vi "test Compare Ports Between Import and Sysdef.vi"(8 "error in":errorcluster, 11 "TestCase in":refnum<class "Refresh.lvclass">) -> (0 "error out":errorcluster, 3 "TestCase out":refnum<class "Refresh.lvclass">)   [LabVIEW 2020, in "Refresh.lvclass"]
uses:
  Refresh.lvclass
  <vilib>/addons/_JKI Toolkits/VI Tester/TestCase.llb/TestCase.lvclass
  niveristand-custom-device-testing-tools/VeriStandTestUtilities/VeriStandTestUtilities.lvlib
  Scripting/AIM/AIM ARINC 429 Scripting.lvlib
  Import/ARINC 429 Import.lvlib
  System Explorer/Implementation/Implementation.lvlib
  C:/Program Files (x86)/National Instruments/LabVIEW 2020/vi.lib/addons/_JKI Toolkits/VI Tester/TestCase.llb/TestCase.lvclass
  C:/git/ni/niveristand-aim-arinc429-custom-device/Source/Custom Device Support/Tests/Unit/Refresh/Refresh.lvclass
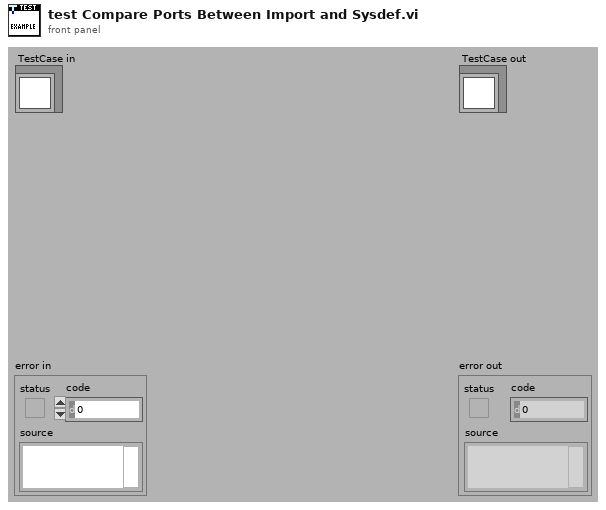
[diagram p1: front panel]
types:
  T1 = typedef "Custom Device API.lvlib/Custom Device Item Ref.ctl" = u64
  T2 = typedef "VS Channels Definition for All Labels on Hardware Channel.ctl" = cluster{"hardware channel":i32, "direction":T3, "labels":T4[], "speed":T9}
  T3 = typedef "Direction.ctl" = enum16{"Rx", "Tx"}
  T4 = typedef "VS Channels Definition for Label.ctl" = cluster{"label (Dec)":u32, "parameters":T5[], "SDI value":u8, "SDI enabled":bool, "transfer type":T8, "create timestamp":bool, "transmit period":u32}
  T5 = typedef "VS Channel Definition for Parameter.ctl" = cluster{"name":string, "unit":string, "Parameter":T6}
  T6 = typedef "Parameter Definition.ctl" = cluster{"start index":i32, "size":i32, "encoding":T7, "signed":bool, "scale multiplier":dbl, "scale offset":dbl, "default value":dbl}
  T7 = typedef "Encoding and Decoding.lvlib/Encoding.ctl" = enum16{"BNR", "BCD", "Discrete"}
  T8 = typedef "Transfer Type.ctl" = enum16{"Scheduled", "Acyclic", "Block", "Strobe"}
  T9 = typedef "Transfer Speed.ctl" = enum16{"LO (12.5 kb/s)", "HI (100 kb/s)"}
  T10 = typedef "AIM ARINC 429 System Explorer.lvlib/Implementation.lvlib/Refresh Listbox.ctl" = cluster{"Item Names":string[], "Item Symbol":T11, "Change Flag":bool}
  T11 = typedef "AIM ARINC 429 System Explorer.lvlib/Implementation.lvlib/Refresh Symbols.ctl" = enum16{"Blank", "Port", "Incoming", "Outgoing", "Label", "Word", "Parameter", "ARINC-429", "Config Files", "Channel Spec", "Item"}
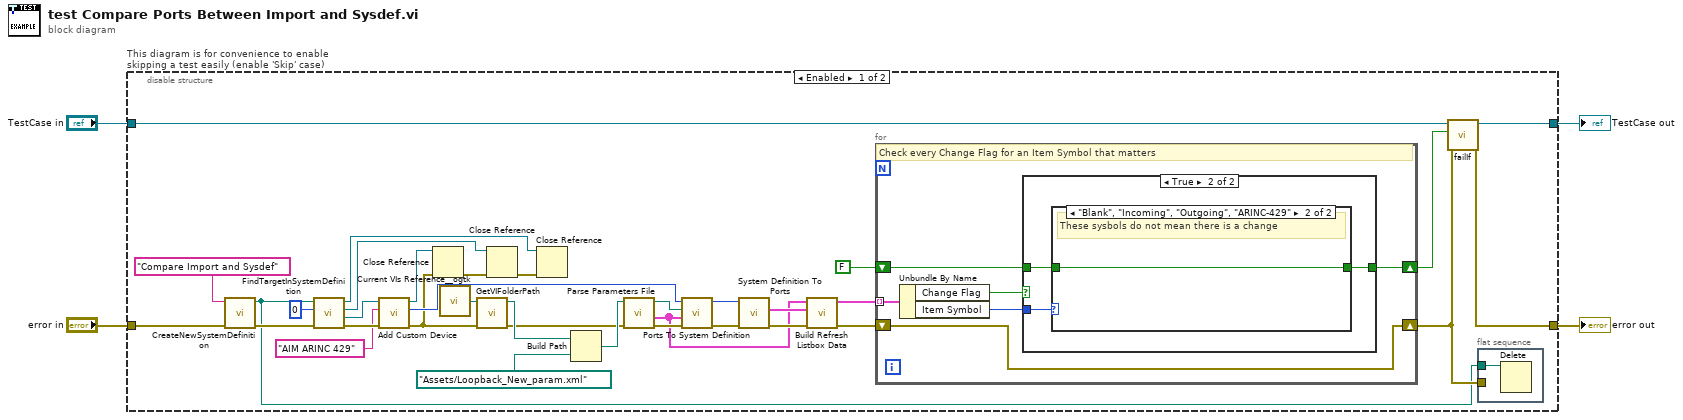
[diagram p0: block diagram]
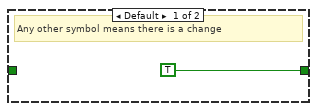
[diagram p3: hidden frame]
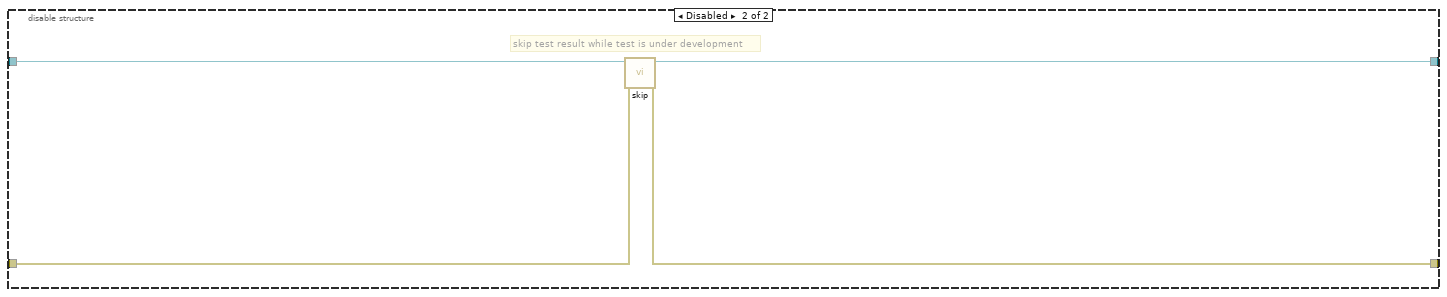
[diagram p4: hidden frame]
diagram:
  n1 = disable-structure "This diagram is for convenience to enable skipping a test easily (enable 'Skip' case)" shown="Enabled" {
    disable-tunnel: "TestCase in" -> [w25 w55]
    disable-tunnel: [w29 w56] -> w1
    disable-tunnel: [w26 w53] -> w3
    disable-tunnel: "error in" -> [w9 w54]
    frame Enabled {
      n2 = call "CreateNewSystemDefinition.vi"("error in"=w9, "System Definition Name"="Compare Import and Sysdef") -> ("error out"=w17:errorcluster, "System Definition Path"=w5:path)  [unwired: 8 in]
      n3 = call "FindTargetInSystemDefinition.vi"("error in"=w17, "target index"=0 ("index"), "system definition path"=w5) -> ("error out"=w20:errorcluster, "Target"=w19:refnum<k24>, "Root"=w13:refnum<k24>, "System Definition"=w12:refnum<k24>)  [unwired: 5 in]
      n4 = call "Add Custom Device.vi"("error in"=w20, "name"="AIM ARINC 429", "target"=w19) -> ("error out"=w8:errorcluster, "AIM ARINC 429 custom device"=w10:T1, "target out"=w16:refnum<k24>)  [unwired: 6 in]
      n5 = Close Reference(reference=w16, error in (no error)=w8) -> (error out=w14:errorcluster)
      n6 = call <userlib>:"Current VIs Reference__ogtk.vi"() -> ("Current VI's reference"=w39:refnum<vi>)  [unwired: 5 in]
      n7 = call "GetVIFolderPath.vi"("error in (no error)"=w8, "VI Reference in"=w39) -> ("error out"=w7:errorcluster, "VI Folder Path out"=w22:path)  [unwired: 8 in]
      n8 = Close Reference(reference=w13, error in (no error)=w14) -> (error out=w15:errorcluster)
      n9 = Close Reference(reference=w12, error in (no error)=w15) -> ()  [unwired: 1 out]
      n10 = Build Path(base path=w22, name or relative path=path "Assets/Loopback_New_param.xml" ("Absolute or Relative Path")) -> (appended path=w11:path)
      n11 = call "Parse Parameters File.vi"("error in"=w7, "path to XML document"=w11) -> ("error out"=w37:errorcluster, "ports"=w32:T2[], "path to XML document out"=w38:path)  [unwired: 7 in]
      n12 = call "Ports To System Definition.vi"("error in"=w37, "ports"=w32, "parameter configuration file path"=w38, "custom device ref"=w10) -> ("error out"=w35:errorcluster, "custom device ref out"=w36:T1)  [unwired: 6 in]
      n13 = call "System Definition To Ports.vi"("error in"=w35, "custom device ref"=w36) -> ("error out"=w34:errorcluster, "ports"=w33:T2[])  [unwired: 7 in, 1 out]
      n14 = call "Build Refresh Listbox Data.vi"("error in"=w34, "new ports"=w33, "current ports"=w32) -> ("error out"=w27:errorcluster, "refresh listbox"=w31:T10[])  [unwired: 7 in]
      n15 = for {
        tunnel: w31 -> [w46] mode=indexing
        shift-right: [w42] -> w28
        shift-left: FALSE -> [w43]
        shift-right: [w41] -> w6
        shift-left: w27 -> [w41]
        # "Check every Change Flag for an Item Symbol that matters"
        n16 = Unbundle By Name(w46) -> ("Change Flag"=w45:bool, "Item Symbol"=w44:T11)
        n17 = case shown="True" w45 {
          tunnel: w44 -> [_ w50]
          tunnel: w43 -> [w47 w49]
          tunnel: [w47 w48] -> w42
          frame False {
          }
          frame True {
            n18 = case shown="\"Blank\", \"Incoming\", \"Outgoing\", \"ARINC-429\"" w50 {
              tunnel: w49 -> [_ w52]
              tunnel: [TRUE w52] -> w48
              frame Default {
                # "Any other symbol means there is a change"
              }
              frame "Blank", "Incoming", "Outgoing", "ARINC-429" {
                # "These sysbols do not mean there is a change"
              }
            }
          }
        }
      }
      n19 = call-dynamic "failIf.vi"("error in (no error)"=w6, "fail"=w28, "TestCase in"=w25) -> ("error out"=w26:errorcluster, "TestCase out"=w29:refnum<class "Refresh.lvclass">)  [unwired: 7 in]
      n20 = flat-sequence {
        tunnel: w6 -> [_]
        tunnel: w5 -> [w40]
        frame #0 {
          n21 = Delete(path (use dialog)=w40) -> ()  [unwired: 4 in, 3 out]
        }
      }
    }
    frame Disabled {
      # "skip test result while test is under development"
      n22 = call <vilib>:"skip.vi"("error in (no error)"=w54, "TestCase in"=w55) -> ("error out"=w53:errorcluster, "TestCase out"=w56:refnum<class "Refresh.lvclass">)  [unwired: 8 in]
    }
  }
  "error out" <- w3
  "TestCase out" <- w1
